vi "dfd_Maxflat Halfband Filter Design.vi"(7 "filter type":enum16{"Lowpass", "Highpass"}(ring), 8 "error IO":errorcluster, 11 "order":i32) -> (0 "error out":errorcluster, 2 "order out":i32, 3 "h out":dbl[](array[numeric]))   [LabVIEW 2017, in "NI_DigFilterLicensed.lvlib"]
uses:
  <vilib>/addons/Digital Filter Design/NI_DigFilterLicensed.lvlib
  <vilib>/Analysis/2dsp.llb/1D Convolution (DBL).vi
  <vilib>/addons/Digital Filter Design/_Misc.llb/dfd_Error Cluster From Error Code (Scalar).vi
  <vilib>/Analysis/polynomials.llb/Create Polynomial From Roots (CDB).vi
  <vilib>/addons/Digital Filter Design/_Misc.llb/dfd_Error Handlers (Multiple).vi
  <vilib>/Analysis/NI_AALPro.lvlib
  <vilib>/addons/Digital Filter Design/NI_DigFilter_Design.lvlib
  <vilib>/addons/Digital Filter Design/NI_DigFilter_Process.lvlib
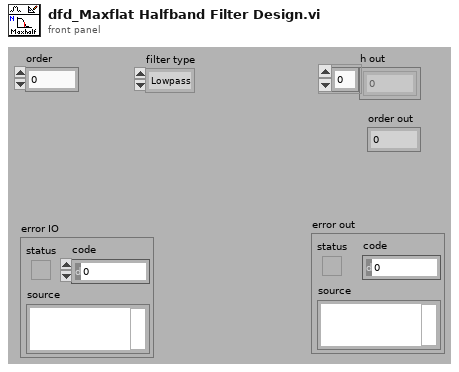
[diagram p1: front panel]
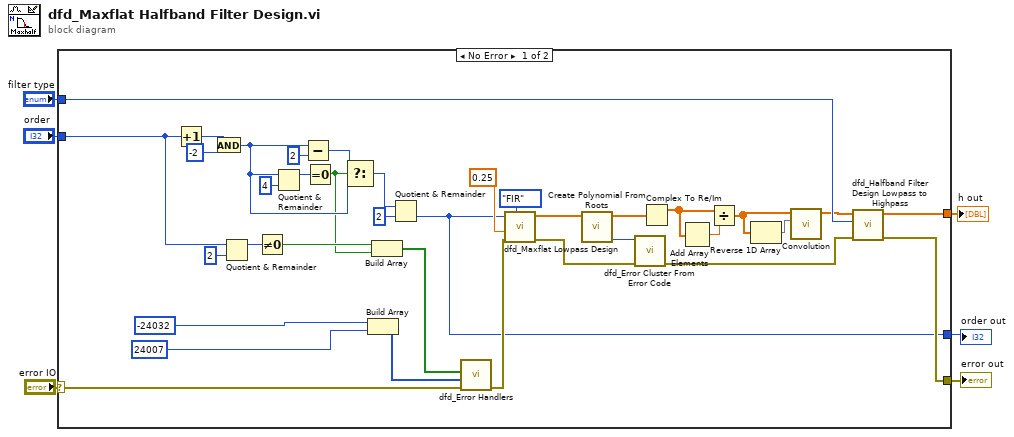
[diagram p0: block diagram]
diagram:
  n1 = case shown="No Error" "error IO" {
    selector: "error IO" -> [w12 w43]
    tunnel: "filter type" -> [w31 _]
    tunnel: [w29 _] -> w5
    tunnel: [w27 w43] -> w4
    tunnel: "order" -> [w19 _]
    tunnel: [w13 _] -> w2
    frame No Error {
      n2 = Increment(x=w19) -> (x+1=w23:i32)
      n3 = And(x=w23, y=-2) -> (x .and. y?=w21:i32)
      n4 = Quotient & Remainder(x=w19, y=2) -> (x-y*floor(x/y)=w32:i32)  [unwired: 1 out]
      n5 = Not Equal To 0?(x=w32) -> (x != 0?=w18:bool)
      n6 = Quotient & Remainder(x=w21, y=4 ("x")) -> (x-y*floor(x/y)=w24:i32)  [unwired: 1 out]
      n7 = Subtract(x=w21, y=2) -> (x-y=w26:i32)
      n8 = Equal To 0?(x=w24) -> (x = 0?=w7:bool)
      n9 = Select(t=w26, s=w7, f=w21) -> (s? t:f=w16:i32)
      n10 = Build Array(-24032 ("ERR_ORDER_ODD"), 24007 ("WRN_ZERO_COEF_REMOVED")) -> (w15:i32[])
      n11 = Build Array(w18, w7) -> (w14:bool[])
      n12 = Quotient & Remainder(x=w16, y=2) -> (floor(x/y)=w13:i32)  [unwired: 1 out]
      n13 = call-poly <vilib>:"dfd_Error Handlers.vi"("error in (no error)"=w12, "error sources"=w15, "condition failed?"=w14) -> ("error out"=w33:errorcluster)  [unwired: 8 out]
      n14 = call <vilib>:"dfd_Maxflat Lowpass Design.vi"("filter type"=enum16{"IIR", "FIR", "Symmetric FIR"}."FIR", "error IO"=w33, "3dB cutoff freq"=0.25, "numerator order"=w13) -> ("error out"=w35:errorcluster, "zeros"=w36:cdb[])  [unwired: 2 in, 4 out]
      n15 = call-poly <vilib>:"Create Polynomial From Roots.vi"("Roots"=w36) -> ("error"=w37:i32, "P(x)"=w39:cdb[])  [unwired: 9 out]
      n16 = call-poly <vilib>:"dfd_Error Cluster From Error Code.vi"("error in (no error)"=w35, "error code (0)"=w37) -> ("error out"=w28:errorcluster)  [unwired: 9 out]
      n17 = Complex To Re/Im(x + iy=w39) -> (x=w38:dbl[])  [unwired: 1 out]
      n18 = Add Array Elements(numeric array=w38) -> (sum=w40:dbl)
      n19 = Divide(x=w38, y=w40) -> (x/y=w34:dbl[])
      n20 = Reverse 1D Array(array=w34) -> (reversed array=w11:dbl[])
      n21 = call-poly <vilib>:"Convolution.vi"("Y"=w11, "X"=w34) -> ("X * Y"=w30:dbl[])  [unwired: 1 in, 8 out]
      n22 = call <vilib>:"dfd_Halfband Filter Design Lowpass to Highpass.vi"("error in (no error)"=w28, "filter type"=w31, "h in"=w30) -> ("error out"=w27:errorcluster, "h out"=w29:dbl[])  [unwired: 7 out]
    }
    frame Error {
    }
  }
  "error out" <- w4
  "h out" <- w5
  "order out" <- w2
